vi "2.vi"() -> ()   [LabVIEW 2019]
panel:
  in  "String":string
  out "Current Case":string
  in  "Vertical Pointer Slide":u32(slide) scale=0.0..10.0
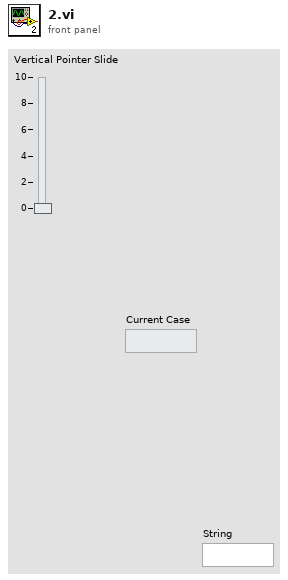
[diagram p1: front panel]
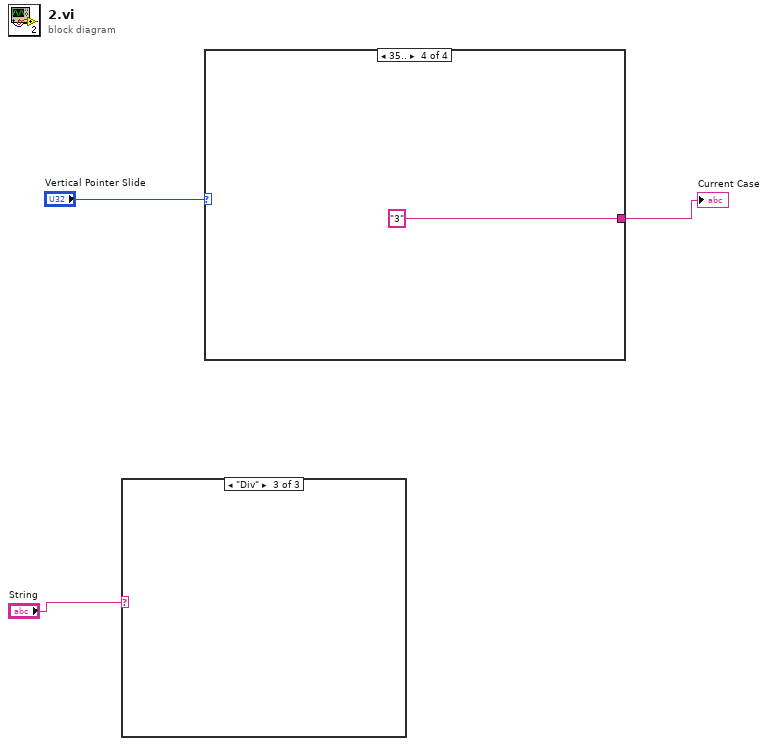
[diagram p0: block diagram]
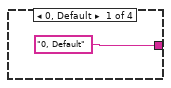
[diagram p4: hidden frame]
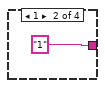
[diagram p5: hidden frame]
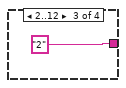
[diagram p6: hidden frame]
diagram:
  n1 = case shown="\"Div\"" "String" {
    frame "Addition" {
    }
    frame "Multiplication" {
    }
    frame "Div" {
    }
  }
  n2 = case shown="35.." "Vertical Pointer Slide" {
    tunnel: ["0, Default" "1" "2" "3"] -> w2
    frame 0, Default {
    }
    frame 1 {
    }
    frame 2..12 {
    }
    frame 35.. {
    }
  }
  "Current Case" <- w2
